vi "Excersise 2.vi"() -> ()   [LabVIEW 2020]
uses:
  <vilib>/addons/Control Design/_Model Construction/Special Model Creation.llb/Special Model Creation SubVI/CD Create PID Parallel Model.vi
  <vilib>/imath/engines/lvmath/Plug In/Control Design/BuiltInFunctions/tf/NIMS_CD_tf(num,den,Ts).vi
  <vilib>/imath/engines/lvmath/Plug In/Control Design/BuiltInFunctions/series/NIMS_CD_series(TF,TF).vi
  <vilib>/imath/engines/lvmath2/RunTimeEngine/NodeEndStatement/NIMS_NodeEndStatement_Output.vi
  <instcachedir>/0/NIMS_NodeEndStatement_Output_53EC0D466D134D7ABD903AC30B43404B.lvgen/NIMS_NodeEndStatement_Output_53EC0D466D134D7ABD903AC30B43404B_009.vi
  <vilib>/imath/engines/lvmath2/RunTimeEngine/ErrorHandling/NIMS_Finalize Error.vi
  <vilib>/addons/Control Design/_Model Interconnection/Model Interconnection.llb/Model Interconnection SubVI/cd_Series (TF and TF).vi
  <vilib>/addons/Control Design/_Model Interconnection/Model Interconnection.llb/Model Interconnection SubVI/cd_Feedback (TF and TF).vi
  <vilib>/addons/Control Design/_Time Response Analysis/Time Response.llb/Time Response subVI/cd_Step Response (Transfer Function).vi
  <vilib>/addons/Control Design/_Frequency Response Analysis/Frequency Response.llb/Frequency Response subVI/cd_Bode (Transfer Function).vi
  <vilib>/addons/Control Design/_Utility/Model Viewer.llb/Model Viewer SubVI/cd_Draw Transfer Function Equation (TF).vi
  <vilib>/addons/Control Design/_Model Construction/NI_CD_Special Model Creation.lvlib
  <vilib>/addons/Control Design/_Model Interconnection/NI_CD_Model Interconnection.lvlib
  <vilib>/addons/Control Design/_Time Response Analysis/NI_CD_Time Response.lvlib
  <vilib>/addons/Control Design/_Frequency Response Analysis/NI_CD_Frequency Response.lvlib
  <vilib>/addons/Control Design/_Utility/NI_CD_Model Viewer.lvlib
panel:
  out "Equation":picture
  in  "J":dbl
  in  "Rm":dbl
  in  "K":dbl
  in  "stop":bool
  out "Step Response Graph":cluster{"time":dbl[], dbl[]}[](graph)
  out "Bode Magnitude":cluster{"W":dbl[], "Magnitude":dbl[]}[](graph)
  in  "Derivative Gain (Kd)":dbl
  in  "Integral Gain (Ki)":dbl
  in  "Proportional Gain (Kp)":dbl=1.0
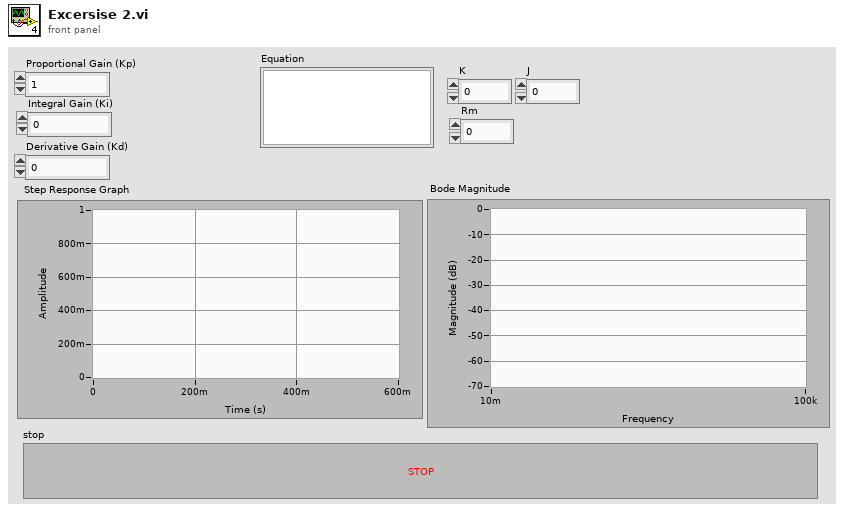
[diagram p1: front panel]
types:
  T1 = typedef "NI_LinSys_Model Typedefs.lvlib/CD Transfer Function Model (MIMO).ctl" = cluster{"properties":T2, "transfer function(s)":T3[][]}
  T2 = typedef "NI_LinSys_Model Typedefs.lvlib/CD General Elements.ctl" = cluster{"Model name":string, "Input names":string[], "Output names":string[], "Input Delays":dbl[], "Output Delays":dbl[], "Sampling Time":dbl, "Notes":string}
  T3 = typedef "NI_LinSys_Model Typedefs.lvlib/CD Transfer Function Model (SISO).ctl" = cluster{"Numerator":dbl[], "Denominator":dbl[], "delay":dbl}
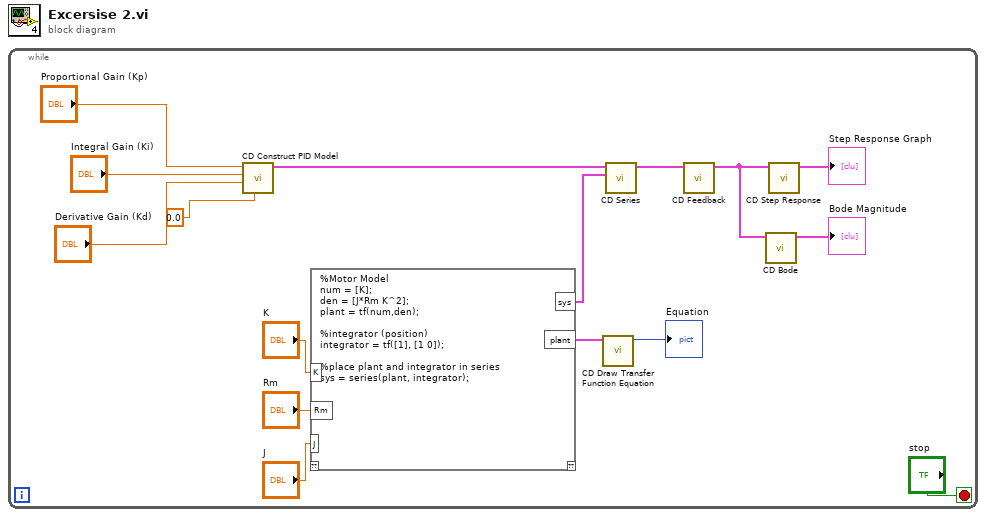
[diagram p0: block diagram]
diagram:
  n1 = while {
    stop <- "stop" stop-if-true
    n2 = call-poly <vilib>:"CD Construct PID Model.vi"("High Frequency Time Constant [s] (Tf)"=0.0, "Derivative Gain (Kd)"="Derivative Gain (Kd)", "Integral Gain (Ki)"="Integral Gain (Ki)", "Proportional Gain (Kp)"="Proportional Gain (Kp)") -> ("Transfer Function Model"=w7:T1)  [unwired: 6 in, 1 out]
    n3 = mathscript code="%Motor Model\nnum = [K];\nden = [J*Rm K^2];\nplant = tf(num,den);\n\n%integrator (position)\nintegrator = tf([1], [1 0]);\n\n%place plant and integrator in series\nsys = series(plant, integrator);"("K"="K", "Rm"="Rm", "J"="J") -> ("plant"=w3:T1, "sys"=w1:T1)  [unwired: 1 in, 1 out]
    n4 = call-poly <vilib>:"CD Draw Transfer Function Equation.vi"("Transfer Function Model"=w3) -> ("Equation"=→"Equation":picture)  [unwired: 8 in, 2 out]
    n5 = call-poly <vilib>:"CD Series.vi"("Model 2"=w1, "Model 1"=w7) -> ("Series Model"=w9:T1)  [unwired: 8 in, 1 out]
    n6 = call-poly <vilib>:"CD Feedback.vi"("Model 1"=w9) -> ("Closed-Loop Model"=w8:T1)  [unwired: 9 in, 1 out]
    n7 = call-poly <vilib>:"CD Bode.vi"("Transfer Function Model"=w8) -> ("Bode Magnitude"=→"Bode Magnitude":cluster{"W":dbl[], "Magnitude":dbl[]}[])  [unwired: 6 in, 4 out]
    n8 = call-poly <vilib>:"CD Step Response.vi"("Transfer Function Model"=w8) -> ("Step Response Graph"=→"Step Response Graph":cluster{"time":dbl[], dbl[]}[])  [unwired: 8 in, 2 out]
  }
